vi "ArmSetGoToTarget.vi"(11 "HeadingToTarget":bool) -> ()   [LabVIEW 2020]
uses:
  ArmGlobal.vi
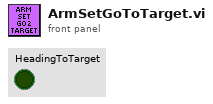
[diagram p1: front panel]
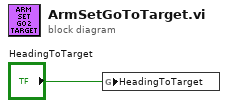
[diagram p0: block diagram]
diagram:
  n1 = global write "ArmGlobal.vi" "HeadingToTarget"("HeadingToTarget") -> ()
